vi "Polyphase Filter_Check Num of Channel.vi"(10 "init":bool, 11 "number of channel":i32) -> (0 "error":i32)   [LabVIEW 2020, in "NI_AAL_Filter.lvlib"]
uses:
  <vilib>/Analysis/NI_AAL_Filter.lvlib
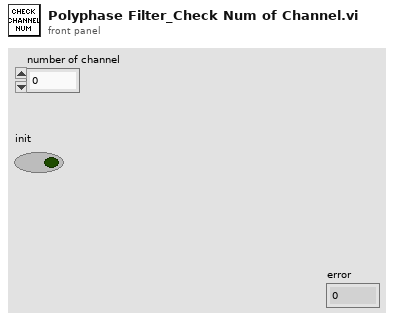
[diagram p1: front panel]
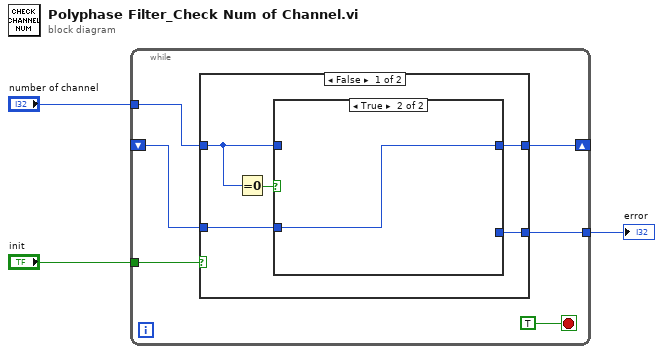
[diagram p0: block diagram]
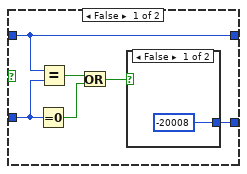
[diagram p2: hidden frame]
diagram:
  n1 = while {
    tunnel: "number of channel" -> [w4]
    shift-right: [w7] -> _
    shift-left: _ -> [w5]
    tunnel: "init" -> [w8]
    tunnel: [w6] -> w2
    stop <- TRUE stop-if-true
    n2 = case shown="False" w8 {
      tunnel: [w10 w23] -> w7
      tunnel: w4 -> [w12 w23]
      tunnel: [w13 _] -> w6
      tunnel: w5 -> [w11 _]
      frame False {
        n3 = Equal To 0?(x=w12) -> (x = 0?=w14:bool)
        n4 = case shown="True" w14 {
          tunnel: [w16 _] -> w13
          tunnel: w12 -> [w15 _]
          tunnel: w11 -> [w20 w22]
          tunnel: [w15 w22] -> w10
          frame False {
            n5 = Equal To 0?(x=w20) -> (x = 0?=w18:bool)
            n6 = Equal?(x=w15, y=w20) -> (x = y?=w19:bool)
            n7 = Or(x=w19, y=w18) -> (x .or. y?=w17:bool)
            n8 = case shown="False" w17 {
              tunnel: [-20008 _] -> w16
              frame False {
              }
              frame True {
              }
            }
          }
          frame True {
          }
        }
      }
      frame True {
      }
    }
  }
  "error" <- w2
